vi "Main - Elapse Time (SubVI).vi"(8 "error in (no error)":errorcluster, 9 "Auto Reset":bool=TRUE, 10 "Init":bool, 11 "Elapsed Time Target":dbl=12.0 format="%0.8f") -> (0 "error out":errorcluster, 2 "Elapse Time":dbl, 3 "Time has Elapsed":bool)   [LabVIEW 2019]
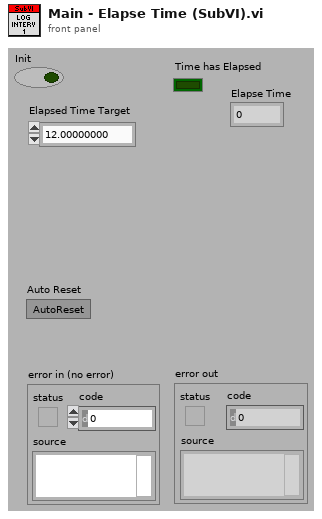
[diagram p1: front panel]
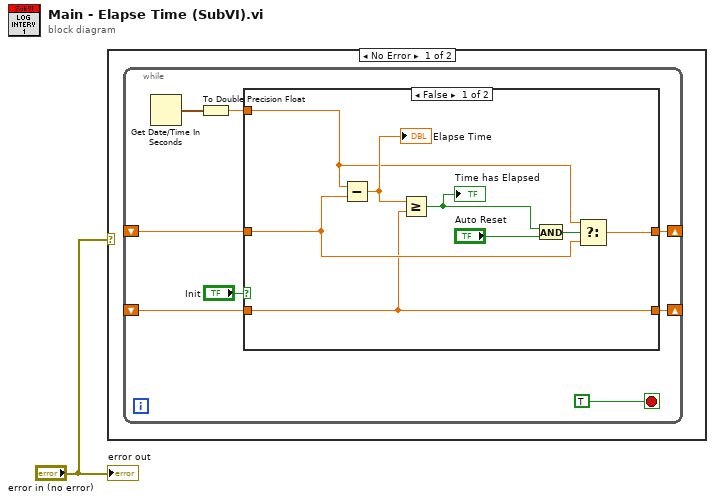
[diagram p0: block diagram]
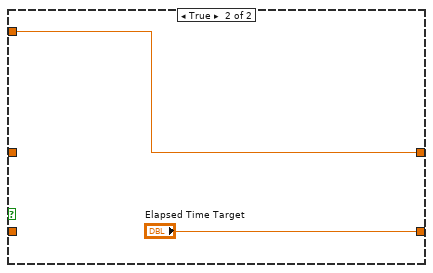
[diagram p2: hidden frame]
diagram:
  n1 = case shown="No Error" "error in (no error)" {
    frame No Error {
      n2 = while {
        shift-right: [w8] -> _
        shift-left: _ -> [w5]
        shift-right: [w3] -> _
        shift-left: _ -> [w2]
        stop <- TRUE stop-if-true
        n3 = Get Date/Time In Seconds() -> (seconds since 1Jan1904=w7:timestamp)
        n4 = To Double Precision Float(number=w7) -> (double precision float=w6:dbl)
        n5 = case shown="False" "Init" {
          tunnel: [w14 w19] -> w8
          tunnel: w6 -> [w12 w19]
          tunnel: w5 -> [w11 _]
          tunnel: [w10 "Elapsed Time Target"] -> w3
          tunnel: w2 -> [w10 _]
          frame False {
            n6 = Subtract(x=w12, y=w11) -> (x-y=w15:dbl)
            "Elapse Time" <- w15
            n7 = Greater Or Equal?(x=w15, y=w10) -> (x >= y?=w17:bool)
            "Time has Elapsed" <- w17
            n8 = And(x=w17, y="Auto Reset") -> (x .and. y?=w13:bool)
            n9 = Select(t=w12, s=w13, f=w11) -> (s? t:f=w14:dbl)
          }
          frame True {
          }
        }
      }
    }
    frame Error {
    }
  }
  "error out" <- "error in (no error)"
